vi "ContourPlot v3.6-dist.vi"() -> ()   [LabVIEW 2024]
uses:
  <vilib>/Utility/file.llb/Read Delimited Spreadsheet (DBL).vi
  <vilib>/Analysis/NI_AALBase.lvlib
panel:
  in  "File name suffix Default: Empty":string(combo)
  out "Ready?":bool=TRUE
  in  "Tab Control 2":enum32{"Contour"}(tab)
  out "Intensity Graph":dbl[][](graph)
  in  "Tab Control":enum32{"IV", "Y curve"}(tab)=enum."Y curve"
  out "IV":cluster{dbl[], "Intensity Graph":dbl[]}(graph)
  in  "intervals":i32=100
  out "Y Histogram":T1(graph)={"X Values"=[0.2739135635, 0.2963500905, 0.3187866175, 0.34122314449999996, 0.36365967149999995, 0.38609619849999993, 0.4085327254999999, 0.4309692524999999, 0.4534057794999999, 0.47584230649999987, 0.49827883349999985, 0.5207153604999999, 0.5431518874999999, 0.5655884144999999, 0.5880249414999998, 0.6104614684999998, 0.6328979954999998, 0.6553345224999998, 0.6777710494999998, 0.7002075764999998, 0.7226441034999997, 0.7450806304999997, 0.7675171574999997, 0.7899536844999997, 0.8123902114999997, 0.8348267384999997, 0.8572632654999996, 0.8796997924999996, 0.9021363194999996, 0.9245728464999996, 0.9470093734999996, 0.9694459004999996, 0.9918824274999996, 1.0143189544999995, 1.0367554814999995, 1.0591920084999995, 1.0816285354999995, 1.1040650624999995, 1.1265015894999995, 1.1489381164999994, 1.1713746434999994, 1.1938111704999994, 1.2162476974999994, 1.2386842244999994, 1.2611207514999994, 1.2835572784999993, 1.3059938054999993, 1.3284303324999993, 1.3508668594999993, 1.3733033864999993, 1.3957399134999993, 1.4181764404999992, 1.4406129674999992, 1.4630494944999992, 1.4854860214999992, 1.5079225484999992, 1.5303590754999992, 1.5527956024999992, 1.5752321294999991, 1.5976686564999991, 1.620105183499999, 1.642541710499999, 1.664978237499999, 1.687414764499999, 1.709851291499999, 1.732287818499999, 1.754724345499999, 1.777160872499999, 1.799597399499999, 1.822033926499999, 1.844470453499999, 1.866906980499999, 1.889343507499999, 1.911780034499999, 1.9342165614999989, 1.9566530884999989, 1.9790896154999988, 2.001526142499999, 2.023962669499999, 2.046399196499999, 2.068835723499999, 2.091272250499999, 2.113708777499999, 2.136145304499999, 2.158581831499999, 2.181018358499999, 2.203454885499999, 2.225891412499999, 2.248327939499999, 2.270764466499999, 2.293200993499999, 2.315637520499999, 2.338074047499999, 2.360510574499999, 2.3829471014999988, 2.4053836284999988, 2.4278201554999987, 2.4502566824999987, 2.4726932094999987, 2.4951297364999987], "Histogram: h(x)"=[1, 0, 0, 0, 0, 0, 0, 0, 0, 0, 0, 0, 0, 0, 0, 0, 0, 0, 1, 0, 0, 0, 0, 0, 0, 0, 0, 0, 0, 0, 0, 0, 0, 0, 1, 0, 0, 0, 0, 0, 0, 0, 0, 1, 1, 0, 0, 0, 0, 0, 0, 0, 0, 0, 0, 0, 0, 0, 0, 0, 0, 0, 2, 0, 0, 0, 0, 0, 0, 0, 3, 7, 3, 8, 12, 17, 22, 35, 58, 64, 95, 151, 176, 250, 309, 406, 525, 769, 931, 994, 1128, 1201, 968, 762, 554, 334, 141, 52, 15, 3]}
  in  "Histogram range":dbl=5.0
  in  "book number":i32=791
  in  "file path (dialog if empty)":path=path "C:/Users/gyue/Desktop/20221209 G22L measurement"
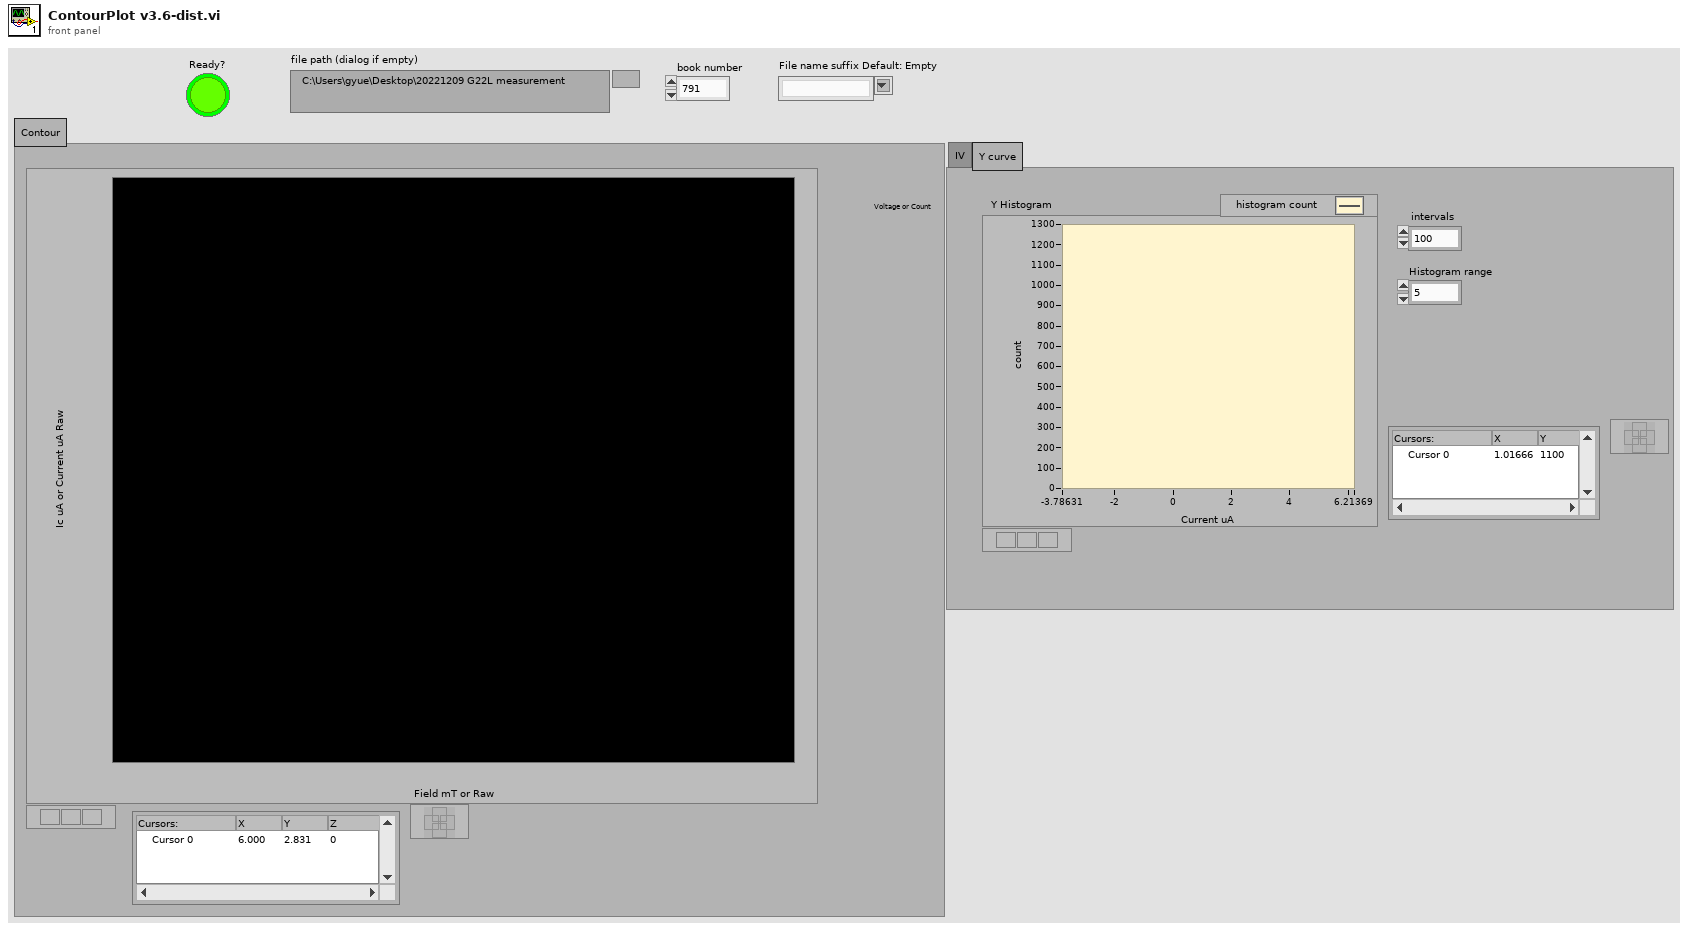
[diagram p1: front panel]
types:
  T1 = cluster{"X Values":dbl[], "Histogram: h(x)":i32[]}
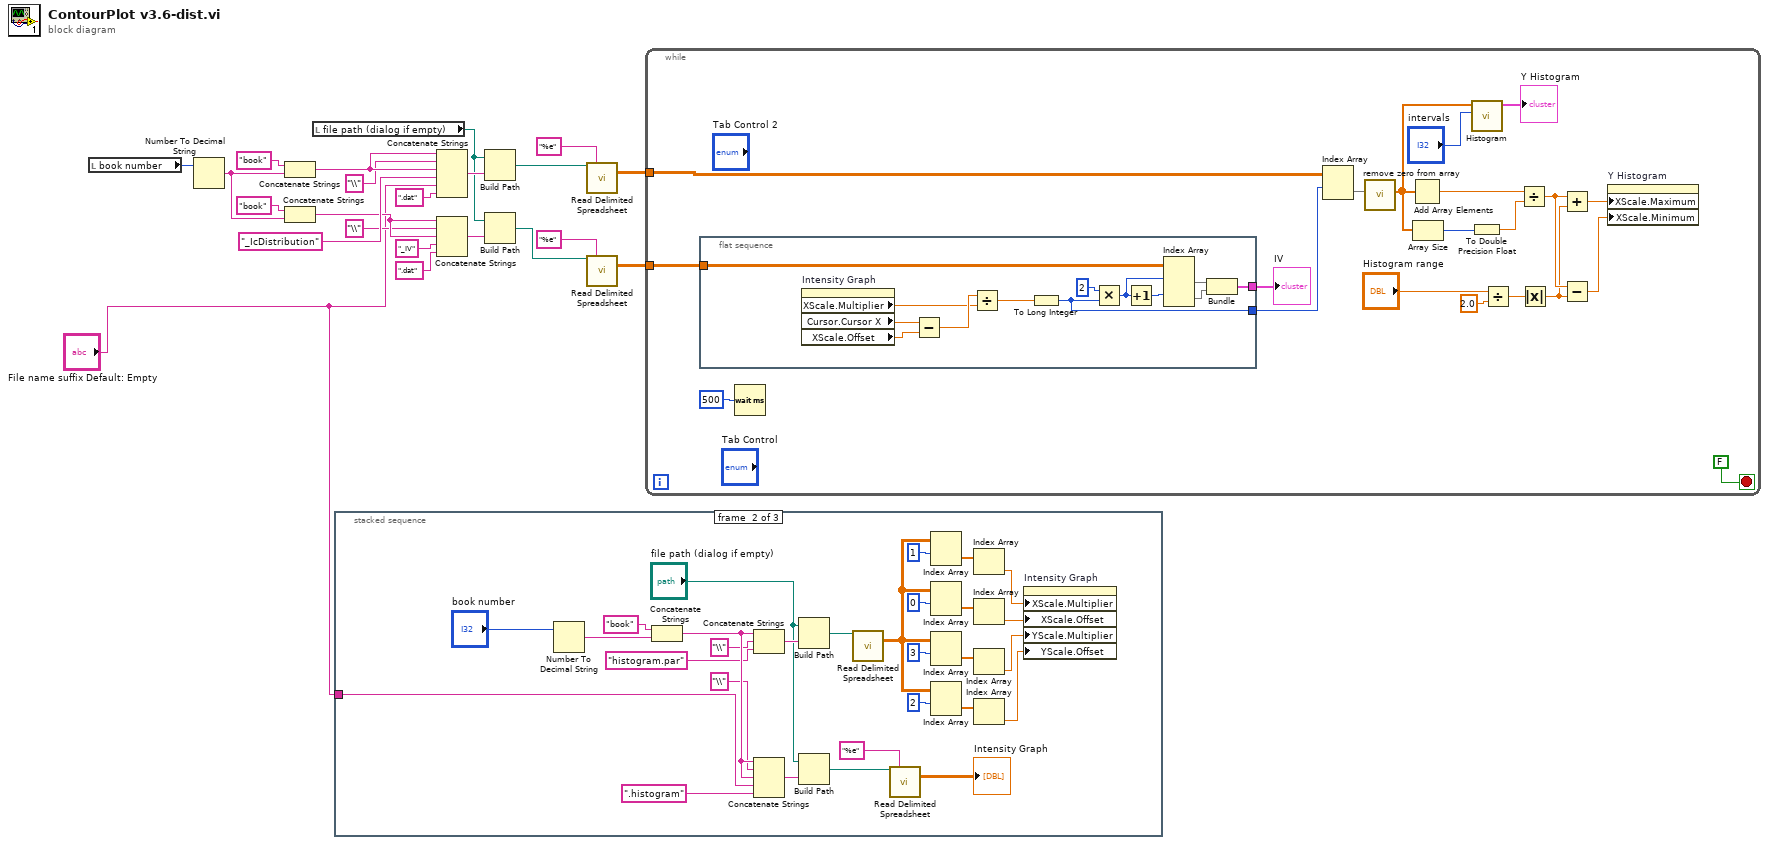
[diagram p0: block diagram]
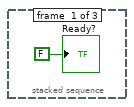
[diagram p2: hidden frame]
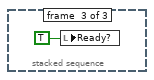
[diagram p3: hidden frame]
diagram:
  n1 = local read "book number"() -> (w18:i32)
  n2 = Number To Decimal String(number=w18) -> (decimal integer string=w5:string)  [unwired: 1 in]
  n3 = Concatenate Strings("book" ("string"), w5) -> (w19:string)
  n4 = Concatenate Strings("book" ("string"), w5) -> (w11:string)
  n5 = local read "file path (dialog if empty)"() -> (w3:path)
  n6 = stacked-sequence {
    tunnel: "File name suffix Default: Empty" -> [_ w24 _]
    frame #0 {
      "Ready?" <- FALSE ("Ready?")
    }
    frame #1 {
      n7 = Number To Decimal String(number="book number") -> (decimal integer string=w48:string)  [unwired: 1 in]
      n8 = Concatenate Strings("book" ("string"), w48) -> (w30:string)
      n9 = Concatenate Strings(w30, "\\" ("string"), "histogram.par" ("string")) -> (w50:string)
      n10 = Concatenate Strings(w30, "\\" ("string"), w30, w24, ".histogram" ("string")) -> (w49:string)
      n11 = Build Path(base path="file path (dialog if empty)", name or relative path=w50) -> (appended path=w51:path)
      n12 = Build Path(base path="file path (dialog if empty)", name or relative path=w49) -> (appended path=w52:path)
      n13 = call-poly <vilib>:"Read Delimited Spreadsheet.vi"("file path (dialog if empty)"=w51) -> ("all rows"=w44:dbl[][])  [unwired: 9 in, 5 out]
      n14 = call-poly <vilib>:"Read Delimited Spreadsheet.vi"("file path (dialog if empty)"=w52, "format (%.3f)"="%e") -> ("all rows"=→"Intensity Graph":dbl[][])  [unwired: 8 in, 5 out]
      n15 = Index Array(array=w44, index (row)=1) -> (element=w40:dbl[])  [unwired: 1 in]
      n16 = Index Array(array=w44, index (row)=0) -> (element=w41:dbl[])  [unwired: 1 in]
      n17 = Index Array(array=w44, index (row)=3) -> (element=w38:dbl[])  [unwired: 1 in]
      n18 = Index Array(array=w44, index (row)=2) -> (element=w39:dbl[])  [unwired: 1 in]
      n19 = Index Array(array=w40) -> (element=w31:dbl)  [unwired: 1 in]
      n20 = Index Array(array=w41) -> (element=w32:dbl)  [unwired: 1 in]
      n21 = Index Array(array=w38) -> (element=w33:dbl)  [unwired: 1 in]
      n22 = Index Array(array=w39) -> (element=w34:dbl)  [unwired: 1 in]
      n23 = property on="Intensity Graph" class="IntGraph (strict)"("XScale.Multiplier"=w31, "XScale.Offset"=w32, "YScale.Multiplier"=w33, "YScale.Offset"=w34) -> ()  [unwired: 2 in, 2 out]
    }
    frame #2 {
      n24 = local write "Ready?"(TRUE ("Ready?")) -> ()
    }
  }
  n25 = Concatenate Strings(w19, "\\" ("string"), w19, "_IcDistribution" ("string"), "File name suffix Default: Empty", ".dat" ("string")) -> (w20:string)
  n26 = Concatenate Strings(w11, "\\" ("string"), w11, "_IV" ("string"), ".dat" ("string")) -> (w12:string)
  n27 = Build Path(base path=w3, name or relative path=w20) -> (appended path=w21:path)
  n28 = Build Path(base path=w3, name or relative path=w12) -> (appended path=w13:path)
  n29 = call-poly <vilib>:"Read Delimited Spreadsheet.vi"("file path (dialog if empty)"=w21, "format (%.3f)"="%e") -> ("all rows"=w22:dbl[][])  [unwired: 8 in, 5 out]
  n30 = call-poly <vilib>:"Read Delimited Spreadsheet.vi"("file path (dialog if empty)"=w13, "format (%.3f)"="%e") -> ("all rows"=w4:dbl[][])  [unwired: 8 in, 5 out]
  n31 = while {
    tunnel: w22 -> [w69]
    tunnel: w4 -> [w66]
    stop <- FALSE stop-if-true
    n32 = flat-sequence {
      tunnel: [w82] -> w73
      tunnel: [w74] -> w70
      tunnel: w66 -> [w79]
      frame #0 {
        n33 = property on="Intensity Graph" class="IntGraph (strict)"() -> ("XScale.Multiplier"=w85:dbl, "Cursor.Cursor X"=w84:dbl, "XScale.Offset"=w83:dbl)  [unwired: 2 in, 2 out]
        n34 = Subtract(x=w84, y=w83) -> (x-y=w86:dbl)
        n35 = Divide(x=w86, y=w85) -> (x/y=w81:dbl)
        n36 = To Long Integer(number=w81) -> (32bit integer=w74:i32)
        n37 = Multiply(x=2, y=w74) -> (x*y=w77:i32)
        n38 = Increment(x=w77) -> (x+1=w76:i32)
        n39 = Index Array(array=w79, index (row) #1=w77, index (row) #2=w76) -> (element #1=w78:dbl[], element #2=w75:dbl[])  [unwired: 2 in]
        n40 = Bundle("all rows"=w78, "all rows"=w75) -> (w82:cluster{"all rows":dbl[], "all rows":dbl[]})  [unwired: 1 in]
      }
    }
    n41 = Wait (ms)(milliseconds to wait=u32 500) -> ()  [unwired: 1 out]
    n42 = Index Array(array=w69, index (row)=w70) -> (element=w55:dbl[])  [unwired: 1 in]
    n43 = call "remove zero from array.vi"("in"=w55) -> ("out"=w54:dbl[])  [unwired: 10 in]
    n44 = Add Array Elements(numeric array=w54) -> (sum=w63:dbl)
    n45 = Array Size(array=w54) -> (size(s)=w62:i32)
    n46 = call <vilib>:"Histogram.vi"("intervals"="intervals", "X"=w54) -> ("Histogram Graph"=→"Y Histogram":T1)  [unwired: 6 in, 3 out]
    n47 = To Double Precision Float(number=w62) -> (double precision float=w61:dbl)
    n48 = Divide(x="Histogram range", y=2.0) -> (x/y=w60:dbl)
    n49 = Divide(x=w63, y=w61) -> (x/y=w58:dbl)
    n50 = Absolute Value(x=w60) -> (abs(x)=w57:dbl)
    n51 = Add(x=w58, y=w57) -> (x+y=w59:dbl)
    n52 = Subtract(x=w58, y=w57) -> (x-y=w56:dbl)
    n53 = property on="Y Histogram" class="XYGraph (strict)"("XScale.Maximum"=w59, "XScale.Minimum"=w56) -> ()  [unwired: 2 in, 2 out]
    "IV" <- w73
  }
